vi "WeightUpdate.vi"(9 "(dE/dOut)(PrevLayerOP)":fxp<+/-,64,32>[](array[numeric]), 10 "Learning Rate":fxp<+/-,64,32>, 11 "weights":fxp<+/-,64,32>[](array[numeric])) -> (2 "dE/dWi":fxp<+/-,64,32>[](array[numeric]) format="%.42g", 3 "w+":fxp<+/-,64,32>[](array[numeric]) format="%.42g")   [LabVIEW 2014]
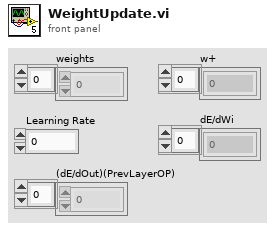
[diagram p1: front panel]
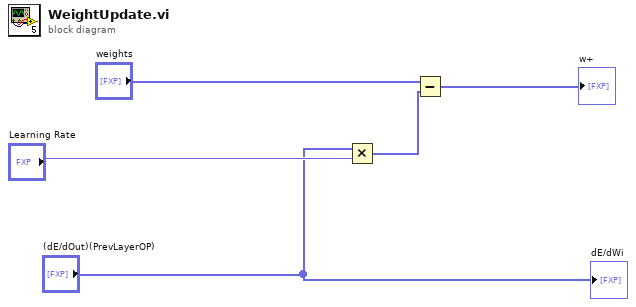
[diagram p0: block diagram]
diagram:
  n1 = Multiply(x="(dE/dOut)(PrevLayerOP)", y="Learning Rate") -> (x*y=w3:fxp<+/-,64,32>[])
  n2 = Subtract(x="weights", y=w3) -> (x-y=→"w+":fxp<+/-,64,32>[])
  "dE/dWi" <- "(dE/dOut)(PrevLayerOP)"
